vi "BuildRelease.vi"() -> ()   [LabVIEW 2014]
uses:
  <vilib>/Utility/traverseref.llb/TRef TravTarget.ctl
  <vilib>/Utility/traverseref.llb/VI Scripting - Traverse.lvlib
panel:
  out "error out":errorcluster
  out "Tab":enum32{"Start", "Building"}(tab)
  in  "Package Build":i32
  in  "AutoInstallAfterBuild":bool
  in  "DeleteRelease":bool
  in  "Output Folder":path=path "C:/OpenGDS" caption="Build folder: C:\\OpenGDS\\1.2.1(Master)"
  in  "LV_Versions":cluster{"LvVersion":string, "Check":bool}[](array[cluster]) caption="LV versions to compile the release for"
  in  "Build":bool
  out "Branch Name":string
  in  "New Version Number":string
  out "Current Version Number":string
  out "Progress":u8(slide) scale=0.0..100.0
  out "Progress":string
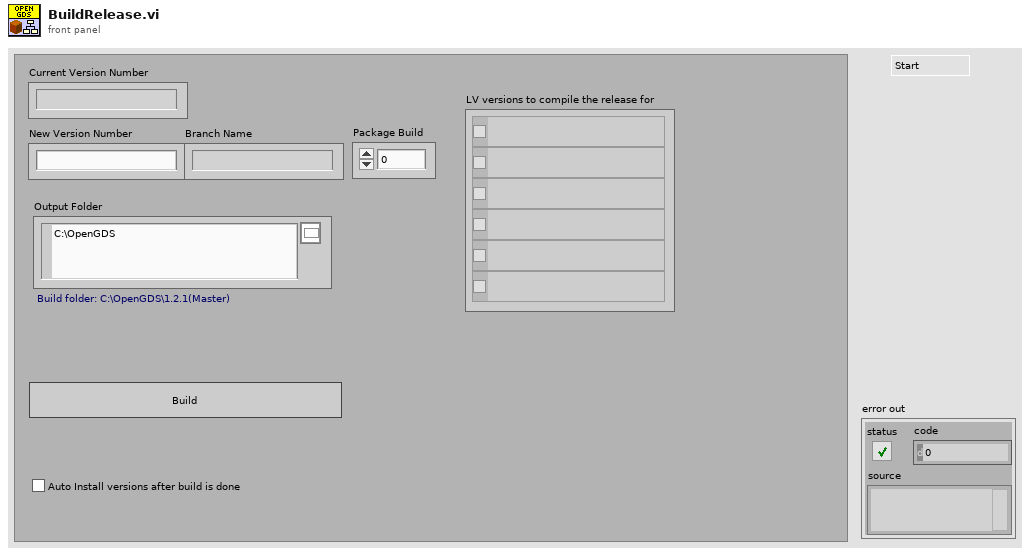
[diagram p1: front panel]
types:
  T1 = cluster{"LvVersion":path[], "BuildPath":path, "SourceFiles":path[], "LvVersion":string[], "SpecFile":path, "IniFiles":path[], "InstallerCopy":path, "VersionName":string, "InstallerFile":path, "ReadMeFile":path, "VIP-File":path, "LogFolder":path}
  T2 = enum32{"invalid OS target", "Mac OS", "Windows 3.1", "Windows 95/NT", "Solaris 1", "Solaris 2", "HP-UX", "PowerMAX", "Linux", "Irix", "Rhapsody", "BeOS", "AIX", "OSF1", "VxWorks", "PharLap", "Carbon", "RTX", "Windows x64", "Linux x64"}
  T3 = enum8{"Enabled", "Disabled", "Disabled and Grayed Out"}
  T4 = typedef "TRef TravTarget.ctl" = enum16{"FP", "BD", "Other"}
  T5 = enum32{"invalid OS target", "Mac OS", "Windows 3.1", "Windows 95/NT", "Solaris 1", "Solaris 2", "HP-UX", "PowerMAX", "Linux", "Irix", "Rhapsody", "BeOS", "AIX", "OSF1", "VxWorks", "PharLap", "Carbon", "RTX", "Windows x64", "Linux x64", "Mac OS X x64"}
  T6 = enum32{"not a typedef", "typedef", "strict typedef", "class private data"}
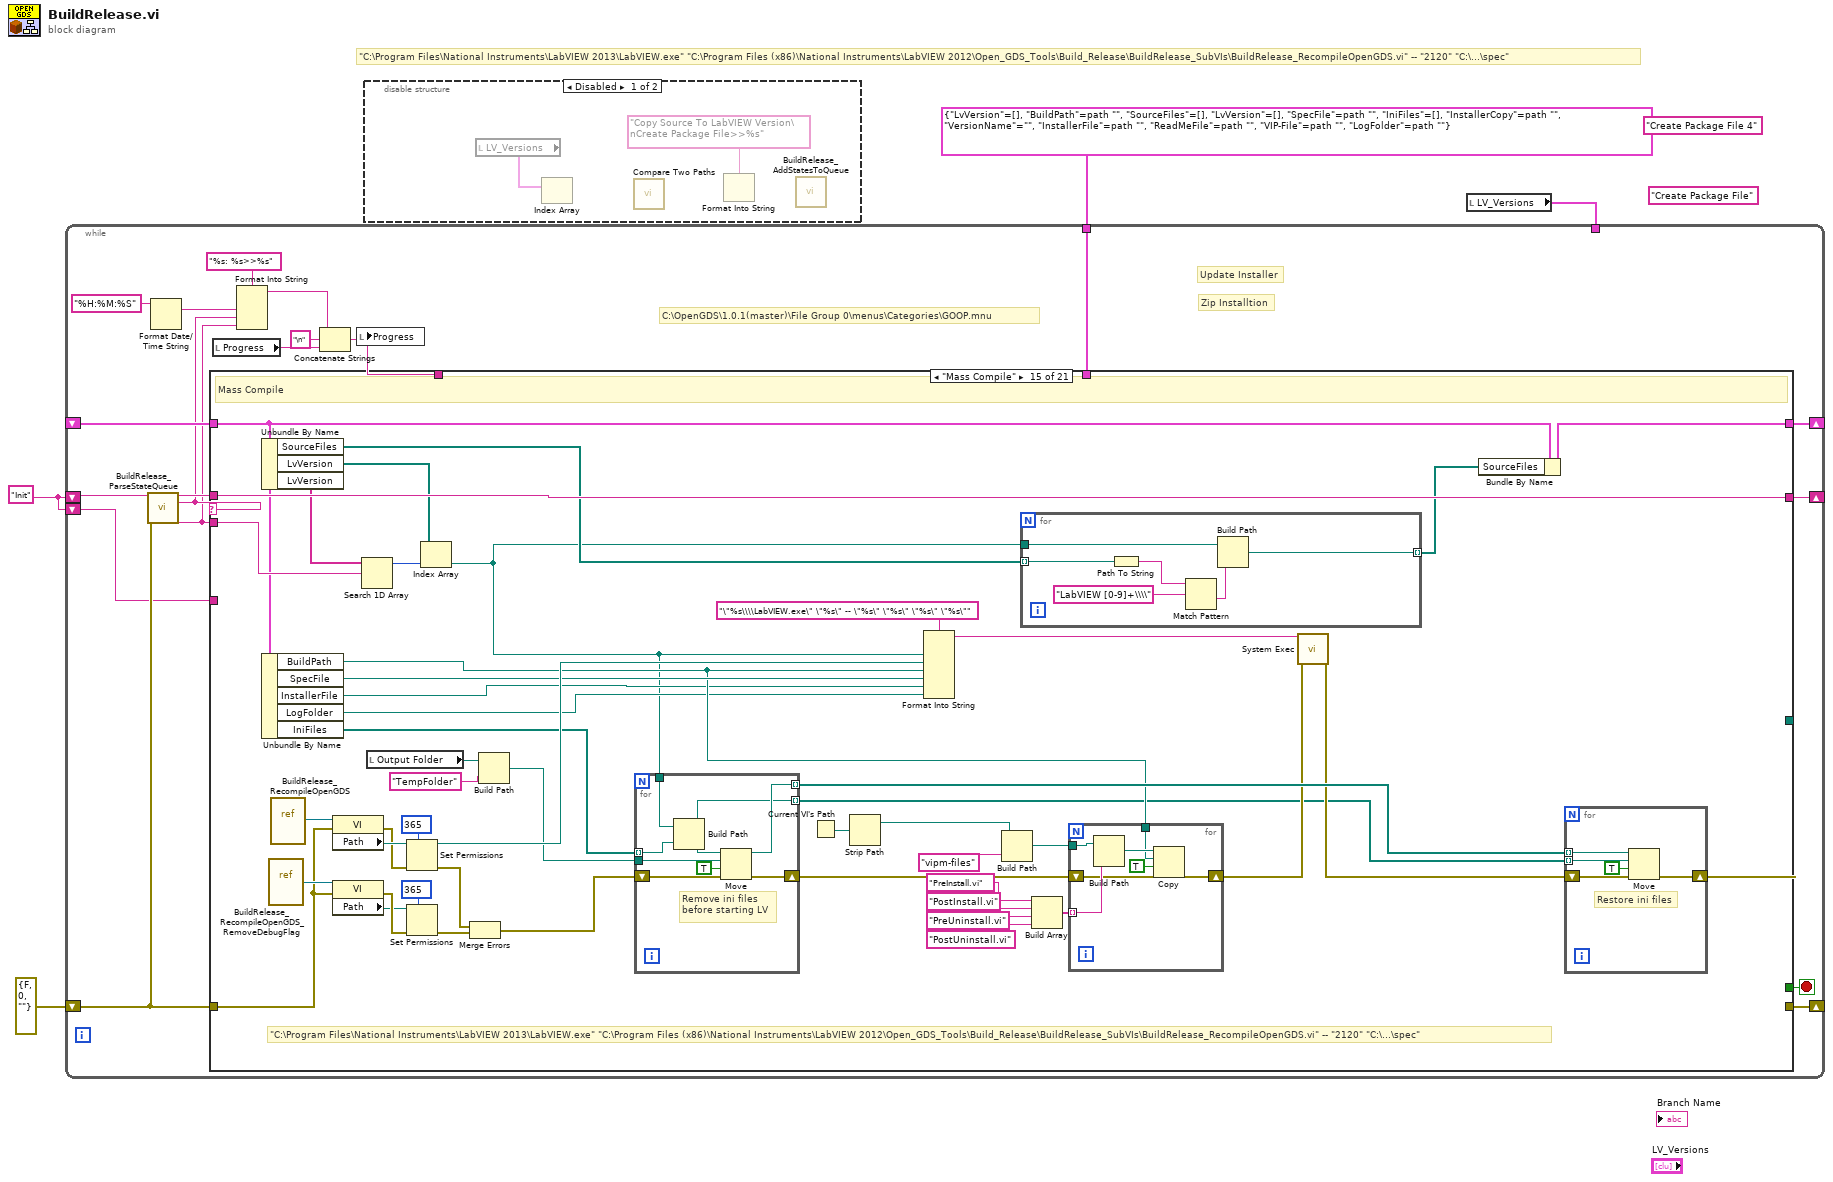
[diagram p0: block diagram]
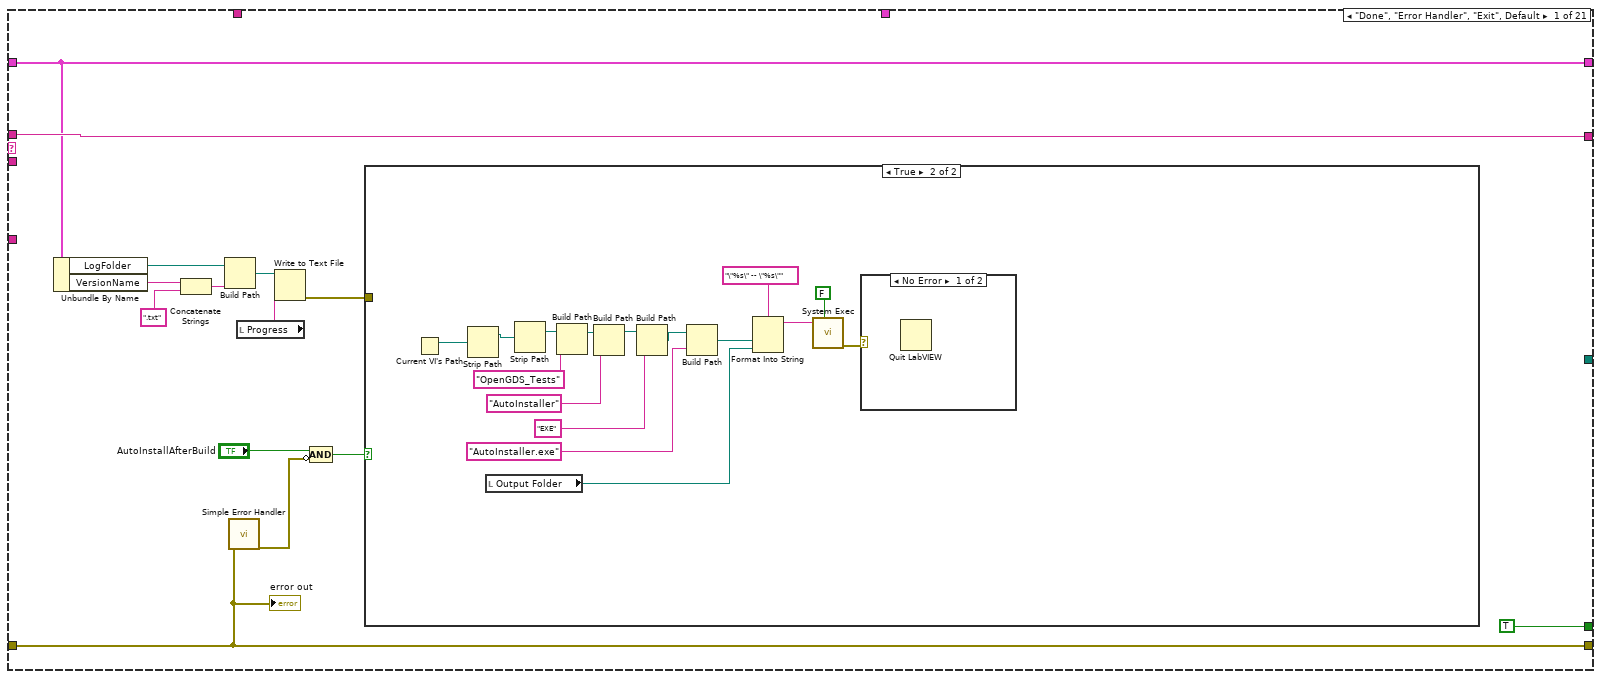
[diagram p3: hidden frame]
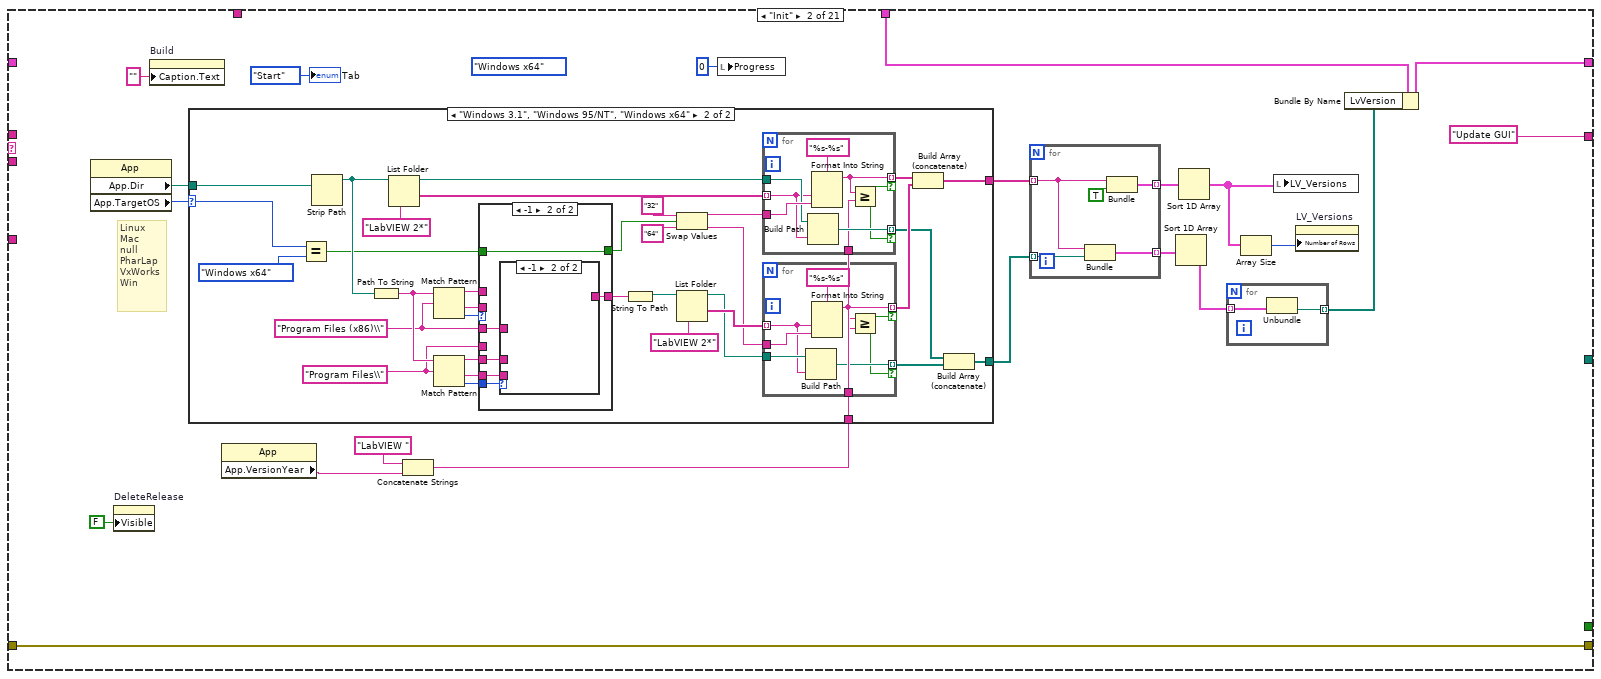
[diagram p6: hidden frame]
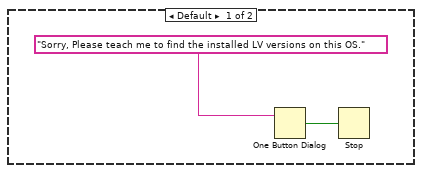
[diagram p7: hidden frame]
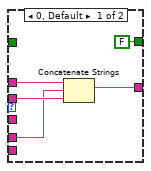
[diagram p8: hidden frame]
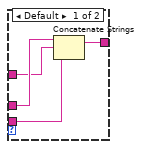
[diagram p9: hidden frame]
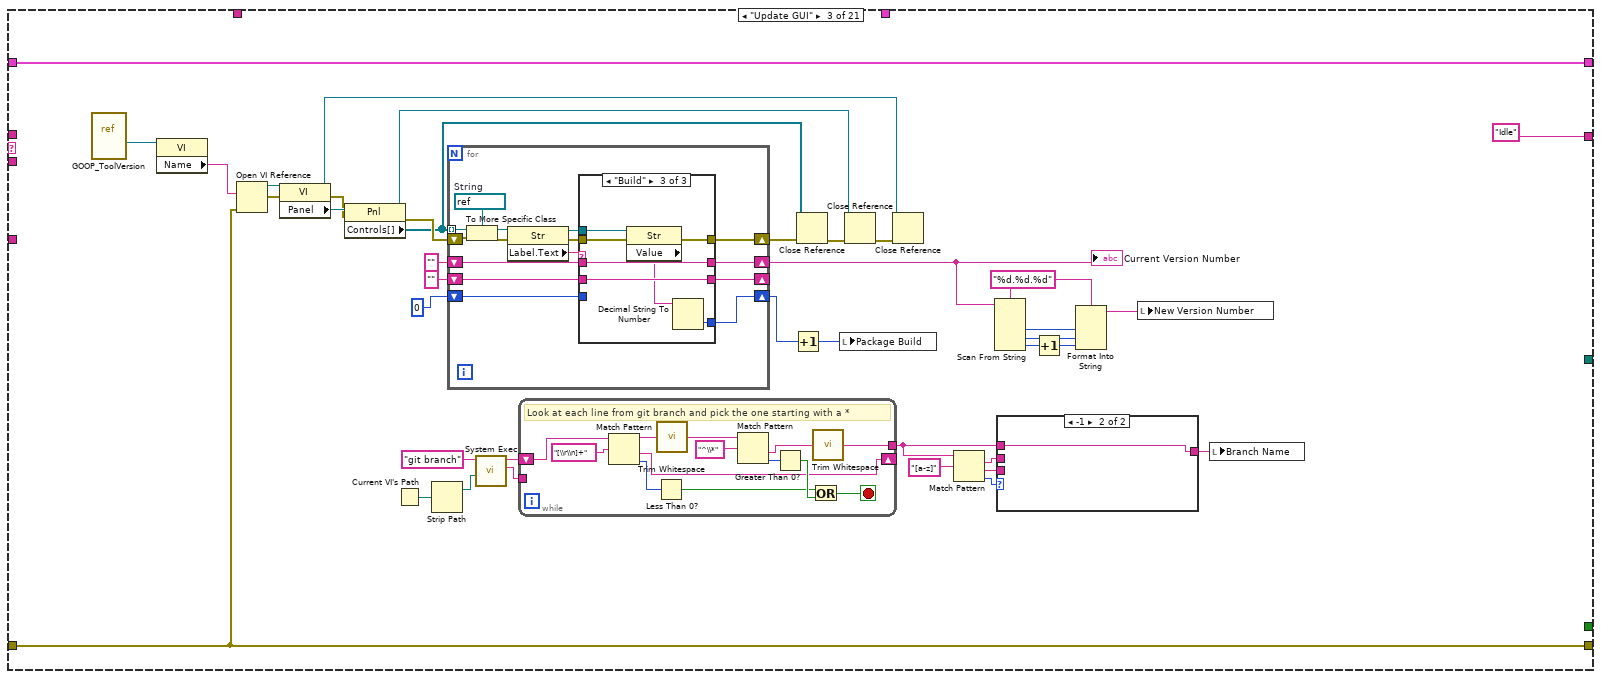
[diagram p10: hidden frame]
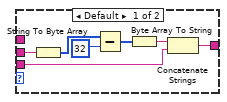
[diagram p11: hidden frame]
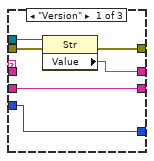
[diagram p12: hidden frame]
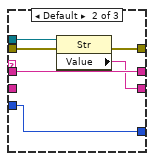
[diagram p13: hidden frame]
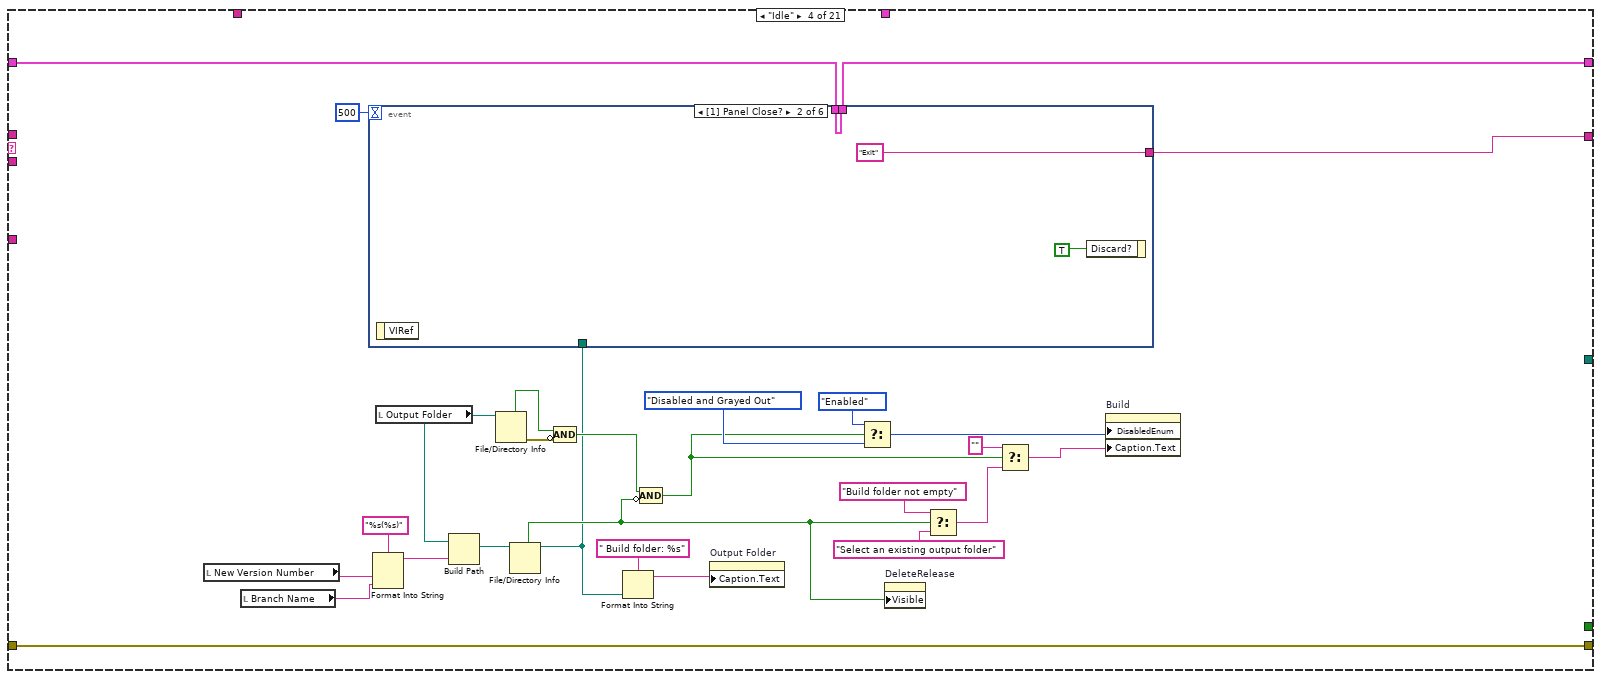
[diagram p14: hidden frame]
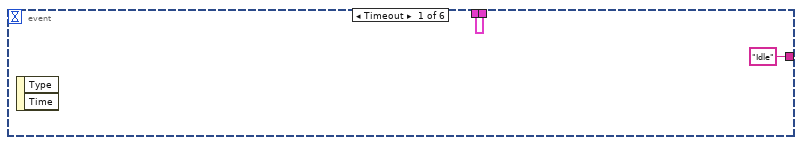
[diagram p15: hidden frame]
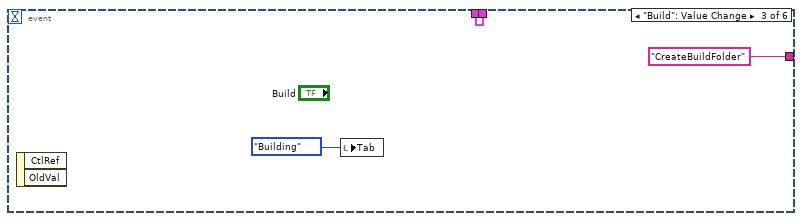
[diagram p16: hidden frame]
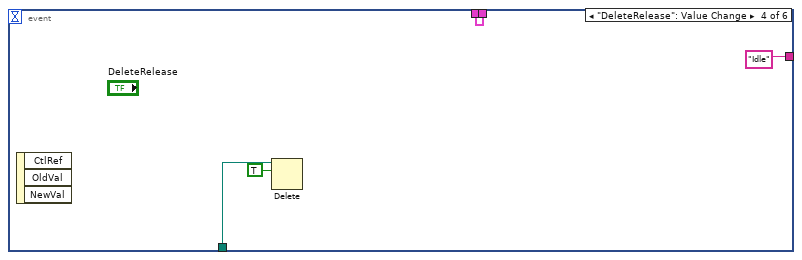
[diagram p17: hidden frame]
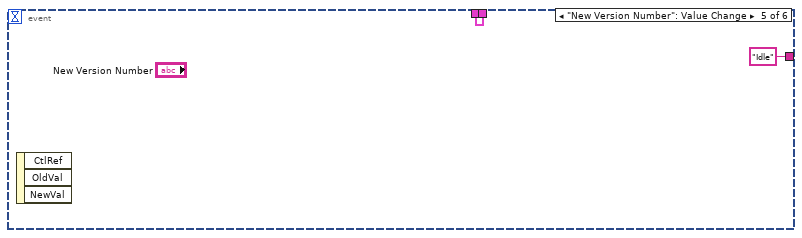
[diagram p18: hidden frame]
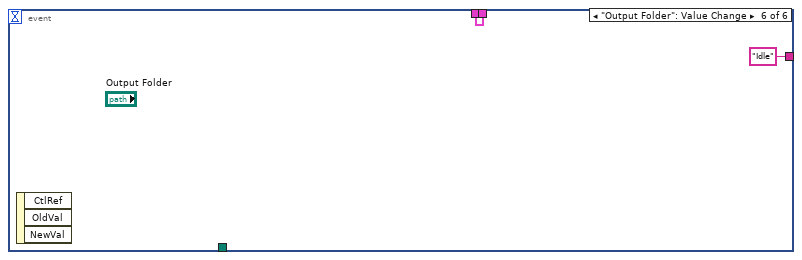
[diagram p19: hidden frame]
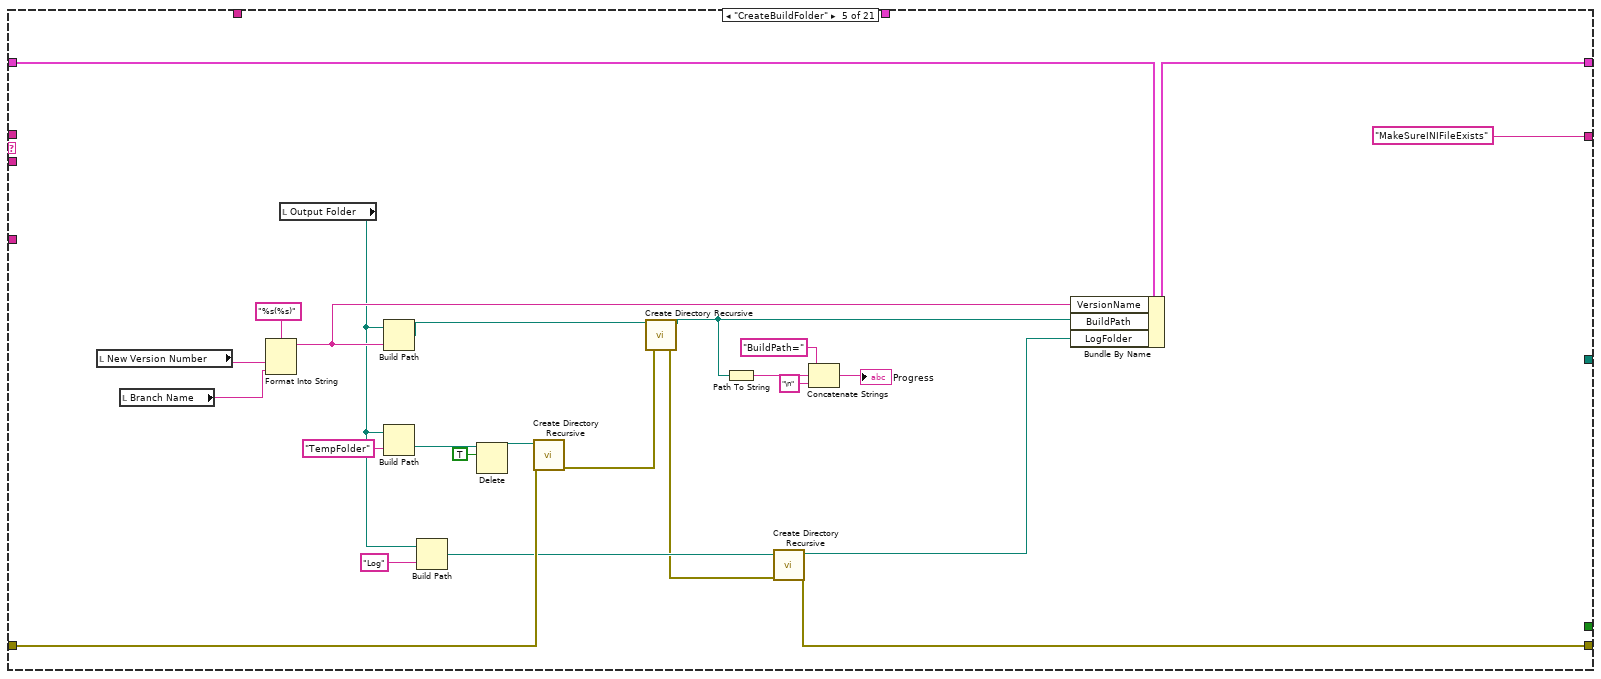
[diagram p20: hidden frame]
diagram:
  (unwired) "Create Package File 4"
  (unwired) "Create Package File"
  w1 = "Init"
  # "\"C:\\Program Files\\National Instruments\\LabVIEW 2013\\LabVIEW.exe\" \"C:\\Program Files (x86)\\National Instruments\\LabVIEW 2012\\Open_GDS_Tools\\Build_Release\\BuildRelease_SubVIs\\BuildRelease_RecompileOpenGDS.vi\" -- \"2120\" \"C:\\...\\spec\""
  n1 = disable-structure shown="Disabled" {
    frame Disabled {
      n2 = local read "LV_Versions"() -> (w5:cluster{"LvVersion":string, "Check":bool}[])
      n3 = Index Array(array=w5) -> ()  [unwired: 1 in, 1 out]
      n4 = call <vilib>:"Compare Two Paths.vi"() -> ()  [unwired: 8 in, 4 out]
      n5 = Format Into String(format string="Copy Source To LabVIEW Version\nCreate Package File>>%s") -> ()  [unwired: 3 in, 2 out]
      n6 = call "BuildRelease_AddStatesToQueue.vi"() -> ()  [unwired: 15 in, 1 out]
    }
    frame Enabled {
    }
  }
  n7 = local read "LV_Versions"() -> (w2:cluster{"LvVersion":string, "Check":bool}[])
  n8 = while {
    shift-right: [w25] -> _
    shift-left: errorcluster {"status"=FALSE, "code"=0, "source"=""} ("error IO") -> [w19]
    shift-right: [w18] -> _
    shift-left: w1 -> [w21]
    shift-right: [w24] -> _
    shift-left: _ -> [w23]
    tunnel: T1 {"LvVersion"=[], "BuildPath"=path "", "SourceFiles"=[], "LvVersion"=[], "SpecFile"=path "", "IniFiles"=[], "InstallerCopy"=path "", "VersionName"="", "InstallerFile"=path "", "ReadMeFile"=path "", "VIP-File"=path "", "LogFolder"=path ""} -> [w22]
    tunnel: w2 -> [_]
    shift-left: w1 -> [w7]
    stop <- w17 stop-if-true
    # "Zip Installtion"
    # "Update Installer"
    # "C:\\OpenGDS\\1.0.1(master)\\File Group 0\\menus\\Categories\\GOOP.mnu"
    n9 = call "BuildRelease_ParseStateQueue.vi"("State Queue"=w21, "Error In (no error)"=w19) -> ("Remaining States"=w20:string, "Current State"=w13:string, "Arguments"=w12:string)  [unwired: 11 in]
    n10 = Format Date/Time String(time format string (%c)="%H:%M:%S") -> (date/time string=w8:string)  [unwired: 2 in]
    n11 = local read "Progress"() -> (w15:string)
    n12 = Format Into String(format string="%s: %s>>%s", w8, w13, w12) -> (resulting string=w11:string)  [unwired: 2 in, 1 out]
    n13 = Concatenate Strings(w11, "\n" ("string"), w15) -> (w14:string)
    n14 = case shown="\"Mass Compile\"" w13 {
      tunnel: w19 -> [w26 w76 w172 w269 w297 w314 w354 w409 w490 w501 w560 w611 w632 w674 w729 w818 w836 w889 w911 w923 w964]
      tunnel: [w26 w76 w172 w269 w289 w313 w341 w397 w483 w500 w561 w611 w632 w658 w756 w803 w835 w877 w910 w930 w964] -> w25
      tunnel: [w37 w75 w189 w270 w308 w327 w340 w393 w492 w504 w559 w603 w631 w657 w755 w819 w826 w872 w913 w920 w963] -> w24
      tunnel: w23 -> [w37 _ w189 w271 w312 w327 w340 w412 w492 w504 w584 w609 w631 w680 w764 w819 w826 w890 w918 w920 w963]
      tunnel: w22 -> [_ w74 _ _ _ _ _ _ _ _ _ _ _ _ _ _ _ _ _ _ _]
      tunnel: w20 -> [w39 _ _ _ _ _ _ _ _ _ _ _ w630 w679 w776 w824 w834 w888 w917 w938 w962]
      tunnel: [w39 "Update GUI" "Idle" w247 "MakeSureINIFileExists" "Update Version Global VI" "Create Package File Spec File" "Add Package Extra Files" "Copy Source To LabVIEW Versions" "Copy Installer VI to Build Folder" "Create Build Process" w604 w630 w679 w776 w824 w834 w888 w917 w938 w962] -> w18
      tunnel: [TRUE _ _ _ _ _ _ _ _ _ _ _ _ _ _ _ _ _ _ _ _] -> w17
      tunnel: w12 -> [_ _ _ _ _ _ _ _ _ _ _ _ _ w633 w774 w822 w830 w879 w906 w932 _]
      tunnel: w14 -> [_ _ _ _ _ _ _ _ _ _ _ _ _ _ _ _ _ _ _ _ _]
      tunnel: w7 -> [_ _ _ _ _ _ _ _ _ _ _ _ _ _ _ _ _ _ _ _ _]
      tunnel: [_ _ _ _ _ _ _ _ _ _ _ _ _ _ _ _ w825 _ _ _ _] -> _
      frame "Done", "Error Handler", "Exit", Default {
        n15 = Unbundle By Name(w37) -> ("LogFolder"=w36:path, "VersionName"=w33:string)
        n16 = Concatenate Strings(w33, ".txt" ("format string")) -> (w32:string)
        n17 = Build Path(base path=w36, name or relative path=w32) -> (appended path=w35:path)
        n18 = call <vilib>:"Simple Error Handler.vi"("error in (no error)"=w26) -> ("error out"=w28:errorcluster)  [unwired: 4 in, 4 out]
        n19 = local read "Progress"() -> (w34:string)
        n20 = Write to Text File(file (use dialog)=w35, text=w34) -> (error out=w27:errorcluster)  [unwired: 2 in, 2 out]
        n21 = Compound Arithmetic op=AND("AutoInstallAfterBuild", invert w28) -> (w29:bool)
        n22 = case shown="True" w29 {
          tunnel: w27 -> [_ _]
          frame False {
          }
          frame True {
            n23 = Current VI's Path() -> (path=w53:path)
            n24 = Strip Path(path=w53) -> (stripped path=w52:path)  [unwired: 1 out]
            n25 = local read "Output Folder"() -> (w42:path)
            n26 = Strip Path(path=w52) -> (stripped path=w51:path)  [unwired: 1 out]
            n27 = Build Path(base path=w51, name or relative path="OpenGDS_Tests") -> (appended path=w49:path)
            n28 = Build Path(base path=w49, name or relative path="AutoInstaller") -> (appended path=w47:path)
            n29 = Build Path(base path=w47, name or relative path="EXE") -> (appended path=w45:path)
            n30 = Build Path(base path=w45, name or relative path="AutoInstaller.exe") -> (appended path=w43:path)
            n31 = Format Into String(format string="\"%s\" -- \"%s\"", w43, w42) -> (resulting string=w54:string)  [unwired: 2 in, 1 out]
            n32 = call <vilib>:"System Exec.vi"("wait until completion? (T)"=FALSE, "command line"=w54) -> ("error out"=w40:errorcluster)  [unwired: 6 in, 3 out]
            n33 = case shown="No Error" w40 {
              frame No Error {
                n34 = Quit LabVIEW() -> ()  [unwired: 1 in]
              }
              frame Error {
              }
            }
          }
        }
        "error out" <- w26
      }
      frame "Init" {
        (unwired) T2."Windows x64" ("y")
        # "Linux\nMac\nnull\nPharLap\nVxWorks\nWin"
        n35 = property class="App"() -> ("App.Dir"=w67:path, "App.TargetOS"=w68:T5)  [unwired: 2 in, 2 out]
        n36 = property on="DeleteRelease" class="Bool"("Visible"=FALSE) -> ()  [unwired: 2 in, 2 out]
        n37 = property on="Build" class="Bool"("Caption.Text"="") -> ()  [unwired: 2 in, 2 out]
        n38 = property class="App"() -> ("App.VersionYear"=w65:string)  [unwired: 2 in, 2 out]
        n39 = Concatenate Strings("LabVIEW " ("pattern"), w65) -> (w64:string)
        n40 = case shown="\"Windows 3.1\", \"Windows 95/NT\", \"Windows x64\"" w68 {
          selector: w68 -> [_ w82]
          tunnel: [_ w114] -> w73
          tunnel: w64 -> [_ w113]
          tunnel: [_ w112] -> w60
          tunnel: w67 -> [_ w81]
          frame Default {
            n41 = One Button Dialog(message="Sorry, Please teach me to find the installed LV versions on this OS.") -> (true=w79:bool)  [unwired: 1 in]
            n42 = Stop(stop? (T)=w79) -> ()
          }
          frame "Windows 3.1", "Windows 95/NT", "Windows x64" {
            w105 = "Program Files\\" ("regular expression")
            w90 = "Program Files (x86)\\" ("regular expression")
            n43 = Equal?(x=w82, y=T2."Windows x64") -> (x = y?=w93:bool)
            n44 = Strip Path(path=w81) -> (stripped path=w108:path)  [unwired: 1 out]
            n45 = Path To String(path=w108) -> (string=w110:string)
            n46 = List Folder(path=w108, pattern="LabVIEW 2*") -> (path out=w84:path, folder names=w101:string[])  [unwired: 2 in, 2 out]
            n47 = Match Pattern(string=w110, regular expression=w90) -> (before substring=w107:string, after substring=w106:string, offset past match=w109:i32)  [unwired: 1 in, 1 out]
            n48 = Match Pattern(string=w110, regular expression=w105) -> (before substring=w92:string, after substring=w91:string, offset past match=w95:i32)  [unwired: 1 in, 1 out]
            n49 = case shown="-1" w109 {
              tunnel: w107 -> [w135 _]
              tunnel: w106 -> [w134 _]
              tunnel: w105 -> [w133 _]
              tunnel: [w132 w136] -> w104
              tunnel: [FALSE w140] -> w100
              tunnel: w95 -> [_ w141]
              tunnel: w93 -> [_ w140]
              tunnel: w92 -> [_ w139]
              tunnel: w91 -> [_ w138]
              tunnel: w90 -> [_ w137]
              frame 0, Default {
                n50 = Concatenate Strings(w135, w133, w134) -> (w132:string)
              }
              frame -1 {
                n51 = case shown="-1" w141 {
                  tunnel: w139 -> [w145 _]
                  tunnel: w138 -> [w144 _]
                  tunnel: w137 -> [w143 _]
                  tunnel: [w142 _] -> w136
                  frame Default {
                    n52 = Concatenate Strings(w145, w143, w144) -> (w142:string)
                  }
                  frame -1 {
                  }
                }
              }
            }
            n53 = String To Path(string=w104) -> (path=w102:path)
            n54 = Swap Values(12:"32" ("format string"), 13:w100, 14:"64" ("format string")) -> (1:w97:string, 3:w87:string)
            n55 = List Folder(path=w102, pattern="LabVIEW 2*") -> (path out=w86:path, folder names=w96:string[])  [unwired: 2 in, 2 out]
            n56 = for {
              tunnel: w101 -> [w127] mode=indexing
              tunnel: w97 -> [w129]
              tunnel: [w125] -> w89 mode=indexing if=w123
              tunnel: w84 -> [w128]
              tunnel: [w126] -> w83 mode=indexing if=w123
              tunnel: w113 -> [w124]
              n57 = Build Path(base path=w128, name or relative path=w127) -> (appended path=w126:path)
              n58 = Format Into String(format string="%s-%s", w127, w129) -> (resulting string=w125:string)  [unwired: 2 in, 1 out]
              n59 = Greater Or Equal?(x=w125, y=w124) -> (x >= y?=w123:bool)
            }
            n60 = for {
              tunnel: w96 -> [w119] mode=indexing
              tunnel: w87 -> [w121]
              tunnel: [w117] -> w88 mode=indexing if=w115
              tunnel: w86 -> [w120]
              tunnel: [w118] -> w85 mode=indexing if=w115
              tunnel: w113 -> [w116]
              n61 = Build Path(base path=w120, name or relative path=w119) -> (appended path=w118:path)
              n62 = Format Into String(format string="%s-%s", w119, w121) -> (resulting string=w117:string)  [unwired: 2 in, 1 out]
              n63 = Greater Or Equal?(x=w117, y=w116) -> (x >= y?=w115:bool)
            }
            n64 = Build Array (concatenate)(w89, w88) -> (w114:string[])
            n65 = Build Array (concatenate)(w83, w85) -> (w112:path[])
          }
        }
        n66 = local write "Progress"(u8 0 ("Progress")) -> ()
        n67 = for {
          tunnel: w73 -> [w149] mode=indexing
          tunnel: [w150] -> w72 mode=indexing
          tunnel: w60 -> [w148] mode=indexing
          tunnel: [w147] -> w58 mode=indexing
          n68 = Bundle(w149, "appended path"=w148) -> (w147:cluster{string, "appended path":path})  [unwired: 1 in]
          n69 = Bundle(w149, "Check"=TRUE) -> (w150:cluster{string, "Check":bool})  [unwired: 1 in]
        }
        n70 = Sort 1D Array(array=w58) -> (sorted array=w57:cluster{string, "appended path":path}[])
        n71 = Sort 1D Array(array=w72) -> (sorted array=w59:cluster{string, "Check":bool}[])
        n72 = for {
          tunnel: w57 -> [w78] mode=indexing
          tunnel: [w77] -> w56 mode=indexing
          n73 = Unbundle(w78) -> ("appended path"=w77:path)  [unwired: 1 out]
        }
        n74 = Array Size(array=w59) -> (size(s)=w71:i32)
        n75 = local write "LV_Versions"(w59) -> ()
        n76 = property on="LV_Versions" class="Arr (strict)"("Number of Rows"=w71) -> ()  [unwired: 2 in, 2 out]
        n77 = Bundle By Name(cluster=w74, "LvVersion"=w56) -> (w75:T1)
        "Tab" <- enum32{"Start", "Building"}."Start" ("Tab")
      }
      frame "Update GUI" {
        w188 = "%d.%d.%d" ("format string")
        n78 = vi-ref <resource>:"GOOP_ToolVersion.vi"() -> (w179:refnum<vi>)
        n79 = property class="VI"(reference=w179) -> ("Name"=w178:string)  [unwired: 1 in, 2 out]
        n80 = Open VI Reference(vi path=w178, error in (no error)=w172) -> (vi reference=w177:refnum<vi>, error out=w176:errorcluster)  [unwired: 4 in]
        n81 = property class="VI"(reference=w177, error in=w176) -> (reference out=w166:refnum<vi>, error out=w173:errorcluster, "Panel"=w175:refnum<vi>)
        n82 = property class="Pnl"(reference=w175, error in=w173) -> (reference out=w168:refnum<vi>, error out=w174:errorcluster, "Controls[]"=w170:refnum<vi>[])
        n83 = Current VI's Path() -> (path=w182:path)
        n84 = Strip Path(path=w182) -> (stripped path=w181:path)  [unwired: 1 out]
        n85 = for {
          tunnel: w170 -> [w224] mode=indexing
          shift-right: [w220] -> w171
          shift-left: w174 -> [w217]
          shift-right: [w216] -> w163
          shift-left: "" ("Value") -> [w215]
          shift-right: [w214] -> _
          shift-left: "" ("Value") -> [w213]
          shift-right: [w211] -> w152
          shift-left: 0 -> [w212]
          w223 = refnum<vi> refnum  # String
          n86 = To More Specific Class(target class=w223, reference=w224, error in=w217) -> (specific class reference=w222:refnum<vi>, error out=w218:errorcluster)
          n87 = property class="Str"(reference=w222, error in=w218) -> (reference out=w221:refnum<vi>, error out=w219:errorcluster, "Label.Text"=w225:string)
          n88 = case shown="\"Build\"" w225 {
            tunnel: w221 -> [w231 w237 w244]
            tunnel: [w229 w236 w243] -> w220
            tunnel: w219 -> [w230 w235 w242]
            tunnel: [w228 w234 w241] -> w216
            tunnel: w215 -> [_ w234 w241]
            tunnel: [w227 w233 w240] -> w214
            tunnel: w213 -> [w227 _ w240]
            tunnel: w212 -> [w226 w232 _]
            tunnel: [w226 w232 w238] -> w211
            frame "Version" {
              n89 = property class="Str"(reference=w231, error in=w230) -> (error out=w229:errorcluster, "Value"=w228:string)  [unwired: 1 out]
            }
            frame Default {
              n90 = property class="Str"(reference=w237, error in=w235) -> (error out=w236:errorcluster, "Value"=w233:string)  [unwired: 1 out]
            }
            frame "Build" {
              n91 = property class="Str"(reference=w244, error in=w242) -> (error out=w243:errorcluster, "Value"=w239:string)  [unwired: 1 out]
              n92 = Decimal String To Number(string=w239) -> (number=w238:i32)  [unwired: 2 in, 1 out]
            }
          }
        }
        "Current Version Number" <- w163
        n93 = call <vilib>:"System Exec.vi"("working directory"=w181, "command line"="git branch") -> ("standard error"=w154:string, "standard output"=w155:string)  [unwired: 6 in, 2 out]
        n94 = while {
          tunnel: [w190] -> w156
          shift-right: [w193] -> _
          shift-left: w155 -> [w197]
          tunnel: w154 -> [_]
          stop <- w196 stop-if-true
          # "Look at each line from git branch and pick the one starting with a *"
          n95 = Match Pattern(string=w197, regular expression="[\\r\\n]+") -> (before substring=w194:string, after substring=w193:string, offset past match=w195:i32)  [unwired: 1 in, 1 out]
          n96 = Less Than 0?(x=w195) -> (x < 0?=w191:bool)
          n97 = call <vilib>:"Trim Whitespace.vi"("string"=w194) -> ("trimmed string"=w202:string)  [unwired: 1 in]
          n98 = Match Pattern(string=w202, regular expression="^\\*") -> (after substring=w200:string, offset past match=w199:i32)  [unwired: 1 in, 2 out]
          n99 = Greater Than 0?(x=w199) -> (x > 0?=w198:bool)
          n100 = Or(x=w191, y=w198) -> (x .or. y?=w196:bool)
          n101 = call <vilib>:"Trim Whitespace.vi"("string"=w200) -> ("trimmed string"=w190:string)  [unwired: 1 in]
        }
        n102 = Increment(x=w152) -> (x+1=w151:i32)
        n103 = Close Reference(reference=w170, error in (no error)=w171) -> (error out=w169:errorcluster)
        n104 = local write "Package Build"(w151) -> ()
        n105 = Close Reference(reference=w168, error in (no error)=w169) -> (error out=w167:errorcluster)
        n106 = Close Reference(reference=w166, error in (no error)=w167) -> ()  [unwired: 1 out]
        n107 = Match Pattern(string=w156, regular expression="[a-z]") -> (match substring=w158:string, after substring=w157:string, offset past match=w160:i32)  [unwired: 1 in, 1 out]
        n108 = Scan From String(format string=w188, input string=w163) -> (output 1=w187:i32, output 2=w186:i32, output 3=w185:i32)  [unwired: 5 in, 3 out]
        n109 = case shown="-1" w160 {
          tunnel: w156 -> [_ w210]
          tunnel: [w203 w210] -> w159
          tunnel: w158 -> [w209 _]
          tunnel: w157 -> [w204 _]
          frame Default {
            n110 = String To Byte Array(string=w209) -> (unsigned byte array=w208:u8[])
            n111 = Subtract(x=w208, y=32) -> (x-y=w206:i32[])
            n112 = Byte Array To String(unsigned byte array=w206) -> (string=w205:string)
            n113 = Concatenate Strings(w205, w204) -> (w203:string)
          }
          frame -1 {
          }
        }
        n114 = Increment(x=w185) -> (x+1=w184:i32)
        n115 = Format Into String(format string=w188, w187, w186, w184) -> (resulting string=w183:string)  [unwired: 2 in, 1 out]
        n116 = local write "New Version Number"(w183) -> ()
        n117 = local write "Branch Name"(w159) -> ()
      }
      frame "Idle" {
        n118 = local read "New Version Number"() -> (w260:string)
        n119 = local read "Branch Name"() -> (w261:string)
        n120 = Format Into String(format string="%s(%s)", w260, w261) -> (resulting string=w258:string)  [unwired: 2 in, 1 out]
        n121 = local read "Output Folder"() -> (w256:path)
        n122 = Build Path(base path=w256, name or relative path=w258) -> (appended path=w257:path)
        n123 = File/Directory Info(path=w256) -> (directory=w267:bool, error out=w268:errorcluster)  [unwired: 1 in, 5 out]
        n124 = File/Directory Info(path=w257) -> (path out=w245:path, directory=w246:bool)  [unwired: 1 in, 5 out]
        n125 = event shown="[1] Panel Close?" {
          selector: _ -> [_ _ _ _ _ _]
          dyn-events: _ -> [_ _ _ _ _ _]
          timeout: 500 -> [_ _ _ _ _ _]
          tunnel: w271 -> [w273 w275 w279 w283 w285 w287]
          tunnel: [w273 w275 w279 w283 w285 w287] -> w270
          tunnel: ["Idle" "Exit" "CreateBuildFolder" "Idle" "Idle" "Idle"] -> w247
          tunnel: w245 -> [_ _ _ w282 _ _]
          event Timeout {
            n126 = event-data() -> ()  [unwired: 1 in, 2 out]
          }
          event Panel Close? {
            n127 = event-data() -> ()  [unwired: 1 in, 1 out]
            n128 = event-data("Discard?"=TRUE) -> ()  [unwired: 1 in, 1 out]
          }
          event "Build": Value Change {
            n129 = event-data() -> ()  [unwired: 1 in, 2 out]
            n130 = local write "Tab"(enum32{"Start", "Building"}."Building" ("Tab")) -> ()
          }
          event "DeleteRelease": Value Change {
            n131 = event-data() -> ()  [unwired: 1 in, 3 out]
            n132 = Delete(path (use dialog)=w282, entire hierarchy (F)=TRUE) -> ()  [unwired: 3 in, 3 out]
          }
          event "New Version Number": Value Change {
            n133 = event-data() -> ()  [unwired: 1 in, 3 out]
          }
          event "Output Folder": Value Change {
            n134 = event-data() -> ()  [unwired: 1 in, 3 out]
          }
        }
        n135 = Compound Arithmetic op=AND(w267, invert w268) -> (w254:bool)
        n136 = Format Into String(format string=" Build folder: %s", w245) -> (resulting string=w249:string)  [unwired: 2 in, 1 out]
        n137 = Compound Arithmetic op=AND(w254, invert w246) -> (w255:bool)
        n138 = property on="Output Folder" class="Path"("Caption.Text"=w249) -> ()  [unwired: 2 in, 2 out]
        n139 = Select(t=T3."Enabled" ("Disabled"), s=w255, f=T3."Disabled and Grayed Out" ("Disabled")) -> (s? t:f=w266:T3)
        n140 = property on="DeleteRelease" class="Bool"("Visible"=w246) -> ()  [unwired: 2 in, 2 out]
        n141 = Select(t="Build folder not empty" ("Caption.Text"), s=w246, f="Select an existing output folder" ("Caption.Text")) -> (s? t:f=w251:string)
        n142 = Select(t="" ("Caption.Text"), s=w255, f=w251) -> (s? t:f=w262:string)
        n143 = property on="Build" class="Bool"("DisabledEnum"=w266, "Caption.Text"=w262) -> ()  [unwired: 2 in, 2 out]
      }
      frame "CreateBuildFolder" {
        n144 = local read "New Version Number"() -> (w310:string)
        n145 = local read "Branch Name"() -> (w311:string)
        n146 = Format Into String(format string="%s(%s)", w310, w311) -> (resulting string=w294:string)  [unwired: 2 in, 1 out]
        n147 = local read "Output Folder"() -> (w293:path)
        n148 = Build Path(base path=w293, name or relative path=w294) -> (appended path=w300:path)
        n149 = Build Path(base path=w293, name or relative path="TempFolder") -> (appended path=w302:path)
        n150 = Build Path(base path=w293, name or relative path="Log") -> (appended path=w291:path)
        n151 = Delete(path (use dialog)=w302, entire hierarchy (F)=TRUE) -> (deleted path=w298:path)  [unwired: 3 in, 2 out]
        n152 = call <vilib>:"Create Directory Recursive.vi"("error in (no error)"=w297, "directory"=w298) -> ("error out"=w296:errorcluster)  [unwired: 3 in, 2 out]
        n153 = call <vilib>:"Create Directory Recursive.vi"("error in (no error)"=w296, "directory"=w300) -> ("error out"=w290:errorcluster, "directory copy"=w299:path)  [unwired: 3 in, 1 out]
        n154 = Path To String(path=w299) -> (string=w306:string)
        n155 = call <vilib>:"Create Directory Recursive.vi"("error in (no error)"=w290, "directory"=w291) -> ("error out"=w289:errorcluster, "directory copy"=w288:path)  [unwired: 3 in, 1 out]
        n156 = Concatenate Strings("BuildPath=" ("string"), w306, "\n" ("string")) -> (→"Progress":string)
        n157 = Bundle By Name(cluster=w312, "VersionName"=w294, "BuildPath"=w299, "LogFolder"=w288) -> (w308:T1)
      }
      frame "MakeSureINIFileExists" {
        # "INI-FILES-GProviders"
        n158 = property class="App"() -> ("App.Dir"=w317:path)  [unwired: 2 in, 2 out]
        n159 = Current VI's Path() -> (path=w325:path)
        n160 = Strip Path(path=w325) -> (stripped path=w324:path)  [unwired: 1 out]
        n161 = Strip Path(path=w324) -> (stripped path=w323:path)  [unwired: 1 out]
        n162 = for {
          shift-right: [w329] -> w315
          shift-left: w317 -> [w330]
          tunnel: string[] ["resource", "Framework", "Providers", "GProviders"] -> [w328] mode=indexing
          n163 = Build Path(base path=w330, name or relative path=w328) -> (appended path=w329:path)
        }
        n164 = Build Path(base path=w323, name or relative path="INI-FILES-GProviders" ("string")) -> (appended path=w321:path)
        n165 = call <vilib>:"Recursive File List.vi"("pattern"="*.ini", "error in (no error)"=w314, "Folder Path"=w321) -> ("error out"=w318:errorcluster, "All Files in Dir"=w319:path[])  [unwired: 4 in, 3 out]
        n166 = for {
          tunnel: w319 -> [w335] mode=indexing
          shift-right: [w331] -> w313
          shift-left: w318 -> [w334]
          tunnel: w315 -> [w332]
          n167 = Copy(8:w334, 9:TRUE ("overwrite (F)"), 10:w332, 11:w335) -> (0:w331:errorcluster)  [unwired: 1 in, 2 out]
        }
      }
      frame "Update Version Global VI" {
        n168 = vi-ref <resource>:"GOOP_ToolVersion.vi"() -> (w356:refnum<vi>)
        n169 = property class="VI"(reference=w356) -> ("Name"=w355:string)  [unwired: 1 in, 2 out]
        n170 = Open VI Reference(vi path=w355, error in (no error)=w354) -> (vi reference=w353:refnum<vi>, error out=w352:errorcluster)  [unwired: 4 in]
        n171 = property class="VI"(reference=w353, error in=w352) -> (reference out=w342:refnum<vi>, error out=w348:errorcluster, "Panel"=w351:refnum<vi>)
        n172 = property class="Pnl"(reference=w351, error in=w348) -> (error out=w349:errorcluster, "Controls[]"=w350:refnum<vi>[])  [unwired: 1 out]
        n173 = local read "New Version Number"() -> (w338:string)
        n174 = local read "Branch Name"() -> (w339:string)
        n175 = local read "Package Build"() -> (w336:i32)
        n176 = for {
          tunnel: w350 -> [w367] mode=indexing
          shift-right: [w363] -> w343
          shift-left: w349 -> [w360]
          tunnel: w338 -> [w359]
          tunnel: w339 -> [w358]
          tunnel: w336 -> [w357]
          w366 = refnum<vi> refnum  # String
          n177 = To More Specific Class(target class=w366, reference=w367, error in=w360) -> (specific class reference=w365:refnum<vi>, error out=w361:errorcluster)
          n178 = property class="Str"(reference=w365, error in=w361) -> (reference out=w364:refnum<vi>, error out=w362:errorcluster, "Label.Text"=w368:string)
          n179 = case shown="\"Build\"" w368 {
            tunnel: w364 -> [w372 w377 w381]
            tunnel: [w370 w375 w380] -> w363
            tunnel: w362 -> [w371 w376 w379]
            tunnel: w359 -> [w369 _ _]
            tunnel: w358 -> [_ _ w378]
            tunnel: w357 -> [_ w374 _]
            frame "Version" {
              n180 = property class="Str"(reference=w372, error in=w371, "Value"=w369) -> (error out=w370:errorcluster)  [unwired: 1 out]
            }
            frame "Build" {
              n181 = Number To Decimal String(number=w374) -> (decimal integer string=w373:string)  [unwired: 1 in]
              n182 = property class="Str"(reference=w377, error in=w376, "Value"=w373) -> (error out=w375:errorcluster)  [unwired: 1 out]
            }
            frame Default {
              n183 = property class="Str"(reference=w381, error in=w379, "Value"=w378) -> (error out=w380:errorcluster)  [unwired: 1 out]
            }
          }
        }
        n184 = invoke class="VI" method="Default Vals.Make Curr Default"(reference=w342, error in=w343) -> (reference out=w345:refnum<vi>, error out=w344:errorcluster)  [unwired: 1 in, 1 out]
        n185 = invoke class="VI" method="Save.Instrument"(reference=w345, error in=w344) -> (reference out=w346:refnum<vi>, error out=w347:errorcluster)  [unwired: 4 in, 4 out]
        n186 = Close Reference(reference=w346, error in (no error)=w347) -> (error out=w341:errorcluster)
      }
      frame "Create Package File Spec File" {
        # "Create The Spec file"
        n187 = Current VI's Path() -> (path=w430:path)
        n188 = Strip Path(path=w430) -> (stripped path=w416:path)  [unwired: 1 out]
        n189 = Build Path(base path=w416, name or relative path="OpenGDS_FileList.txt") -> (appended path=w426:path)
        n190 = Build Path(base path=w416, name or relative path="vipm-files") -> (appended path=w415:path)
        n191 = property class="App"() -> ("App.Dir"=w427:path)  [unwired: 2 in, 2 out]
        n192 = Read from Text File(file (use dialog)=w426, error in=w409) -> (text=w425:string, error out=w408:errorcluster)  [unwired: 2 in, 2 out]
        n193 = call <vilib>:"Trim Whitespace.vi"("string"=w425) -> ("trimmed string"=w424:string)  [unwired: 1 in]
        n194 = Build Path(base path=w415, name or relative path="vipm_spec_template.txt") -> (appended path=w419:path)
        n195 = Spreadsheet String To Array(delimiter (Tab)="\n", format string="%s", spreadsheet string=w424, array type (2D Dbl)=string[] []) -> (array=w420:string[])
        n196 = Read from Text File(file (use dialog)=w419, error in=w408) -> (text=w388:string, error out=w407:errorcluster)  [unwired: 2 in, 2 out]
        n197 = for {
          tunnel: w427 -> [w451]
          tunnel: w420 -> [w452] mode=indexing
          tunnel: [w446] -> w405 mode=concatenating
          n198 = Build Path(base path=w451, name or relative path=w452) -> (appended path=w450:path)
          n199 = File/Directory Info(path=w450) -> (path out=w447:path, directory=w448:bool, error out=w449:errorcluster)  [unwired: 1 in, 4 out]
          n200 = case shown="No Error" w449 {
            selector: w449 -> [w454 _]
            tunnel: w448 -> [w456 _]
            tunnel: w447 -> [w455 _]
            tunnel: [w453 _] -> w446
            frame No Error {
              n201 = case shown="False" w456 {
                tunnel: w455 -> [w458 w461]
                tunnel: w454 -> [_ w460]
                tunnel: [w457 w459] -> w453
                frame False {
                  n202 = Build Array(w458) -> (w457:path[])
                }
                frame True {
                  n203 = call <vilib>:"Recursive File List.vi"("error in (no error)"=w460, "Folder Path"=w461) -> ("All Files in Dir"=w459:path[])  [unwired: 5 in, 4 out]
                }
              }
            }
            frame Error {
            }
          }
        }
        n204 = local read "New Version Number"() -> (w386:string)
        n205 = Format Into String(format string=".%d", initial string=w386, "Package Build") -> (resulting string=w383:string)  [unwired: 1 in, 1 out]
        n206 = Search and Replace String(input string=w388, search string="<version>", replace string=w383) -> (result string=w389:string)  [unwired: 5 in, 3 out]
        n207 = Array Size(array=w405) -> (size(s)=w391:i32)
        n208 = stacked-sequence {
          tunnel: w391 -> [_]
          tunnel: [w431] -> w390
          frame #0 {
            n209 = Format Date/Time String(time format string (%c)="%H:%M: ") -> (date/time string=w431:string)  [unwired: 2 in]
          }
        }
        n210 = Bundle By Name(cluster=w412, "SourceFiles"=w405) -> (w406:T1)
        n211 = Format Into String(format string="%d\n", initial string=w389, w391) -> (resulting string=w417:string)  [unwired: 1 in, 1 out]
        n212 = Format Into String(format string="Files:%d", initial string=w390, w391) -> (resulting string=w399:string)  [unwired: 1 in, 1 out]
        n213 = local read "Progress"() -> (w402:string)
        n214 = for {
          tunnel: w405 -> [w439] mode=indexing
          shift-right: [w441] -> w394
          shift-left: w417 -> [w445]
          tunnel: [w434] -> w382 mode=indexing if=w433
          i -> [w443]
          n215 = Path To String(path=w439) -> (string=w440:string)
          n216 = Strip Path(path=w439) -> (name=w438:string)  [unwired: 1 out]
          n217 = Match Pattern(string=w440, regular expression="LabVIEW [0-9]+[\\\\/]") -> (after substring=w435:string)  [unwired: 1 in, 3 out]
          n218 = Match Pattern(string=w438, regular expression="^GOOP_[A-Za-z]+.ini$") -> (offset past match=w436:i32)  [unwired: 1 in, 3 out]
          n219 = Format Into String(format string="File %d=\"%s\"\n", initial string=w445, w443, w435) -> (resulting string=w441:string)  [unwired: 1 in, 1 out]
          n220 = String To Path(string=w435) -> (path=w434:path)
          n221 = Greater Or Equal To 0?(x=w436) -> (x >= 0?=w433:bool)
        }
        n222 = Concatenate Strings(w399, "\n" ("string"), w402) -> (w403:string)
        n223 = Unbundle By Name(w406) -> ("BuildPath"=w411:path)
        n224 = local write "Progress"(w403) -> ()
        n225 = Build Path(base path=w411, name or relative path="spec") -> (appended path=w410:path)
        n226 = Write to Text File(file (use dialog)=w410, text=w394, error in=w407) -> (error out=w398:errorcluster)  [unwired: 1 in, 2 out]
        n227 = local read "Output Folder"() -> (w395:path)
        n228 = Build Path(base path=w395, name or relative path="spec_File.txt") -> (appended path=w392:path)
        n229 = Bundle By Name(cluster=w406, "IniFiles"=w382, "SpecFile"=w392) -> (w393:T1)
        n230 = Write to Text File(file (use dialog)=w392, text=w394, error in=w398) -> (error out=w397:errorcluster)  [unwired: 1 in, 2 out]
      }
      frame "Add Package Extra Files" {
        # "Copy extra files"
        n231 = Current VI's Path() -> (path=w496:path)
        n232 = Strip Path(path=w496) -> (stripped path=w494:path)  [unwired: 1 out]
        n233 = property class="App"() -> ("App.Dir"=w488:path)  [unwired: 2 in, 2 out]
        n234 = Build Path(base path=w494, name or relative path="vipm-files") -> (appended path=w471:path)
        n235 = Unbundle By Name(w492) -> ("BuildPath"=w477:path)
        n236 = Build Path(base path=w488, name or relative path="LICENSE") -> (appended path=w486:path)
        n237 = Build Path(base path=w471, name or relative path="icon.bmp") -> (appended path=w491:path)
        n238 = Build Path(base path=w471, name or relative path="PreInstall.vi") -> (appended path=w475:path)
        n239 = Build Path(base path=w471, name or relative path="PostInstall.vi") -> (appended path=w469:path)
        n240 = Build Path(base path=w471, name or relative path="PreUninstall.vi") -> (appended path=w468:path)
        n241 = Build Path(base path=w471, name or relative path="PostUninstall.vi") -> (appended path=w467:path)
        n242 = Copy(8:w490, 9:TRUE ("overwrite (F)"), 10:w477, 11:w491) -> (0:w489:errorcluster)  [unwired: 1 in, 2 out]
        n243 = Copy(8:w489, 10:w477, 11:w486) -> (0:w481:errorcluster)  [unwired: 2 in, 2 out]
        n244 = Copy(8:w481, 9:TRUE ("overwrite (F)"), 10:w477, 11:w475) -> (0:w480:errorcluster)  [unwired: 1 in, 2 out]
        n245 = Copy(8:w480, 9:TRUE ("overwrite (F)"), 10:w477, 11:w469) -> (0:w479:errorcluster)  [unwired: 1 in, 2 out]
        n246 = Copy(8:w479, 9:TRUE ("overwrite (F)"), 10:w477, 11:w468) -> (0:w478:errorcluster)  [unwired: 1 in, 2 out]
        n247 = Copy(8:w478, 9:TRUE ("overwrite (F)"), 10:w477, 11:w467) -> (0:w470:errorcluster)  [unwired: 1 in, 2 out]
        n248 = Build Path(base path=w477, name or relative path="File Group 0") -> (appended path=w484:path)
        n249 = Create Folder(path (use dialog)=w484, error in=w470) -> (error out=w483:errorcluster)  [unwired: 1 in, 2 out]
      }
      frame "Copy Source To LabVIEW Versions" {
        # "Copy source files to all LV version selected"
        n250 = Unbundle By Name(w504) -> ("SourceFiles"=w499:path[], "LvVersion"=w502:path[])
        n251 = local read "LV_Versions"() -> (w503:cluster{"LvVersion":string, "Check":bool}[])
        n252 = property class="App"() -> ("App.Dir"=w498:path)  [unwired: 2 in, 2 out]
        n253 = for {
          tunnel: w503 -> [w515] mode=indexing
          tunnel: w502 -> [w507] mode=indexing
          shift-right: [w510] -> w500
          shift-left: w501 -> [w511]
          tunnel: w499 -> [w509]
          tunnel: w498 -> [w508]
          i -> [w513]
          n254 = Unbundle(w515) -> ("LvVersion"=w506:string, "Check"=w505:bool)
          n255 = Greater Than 0?(x=w513) -> (x > 0?=w512:bool)
          n256 = And(x=w505, y=w512) -> (x .and. y?=w514:bool)
          n257 = case shown="True" w514 {
            tunnel: w511 -> [w516 w526]
            tunnel: [w516 w525] -> w510
            tunnel: w509 -> [_ w529]
            tunnel: w508 -> [_ w528]
            tunnel: w507 -> [_ w527]
            tunnel: w506 -> [_ w519]
            frame False {
            }
            frame True {
              n258 = for {
                N -> [w537]
                tunnel: w529 -> [w550] mode=indexing
                tunnel: w528 -> [w551]
                tunnel: w527 -> [w549]
                shift-right: [w530] -> w525
                shift-left: w526 -> [w546]
                i -> [w538]
                stop <- w530 stop-if-true
                n259 = call <vilib>:"Compare Two Paths.vi"("Path 2"=w550, "Path 1"=w551) -> ("Relative Path from 1 to 2"=w548:path)  [unwired: 6 in, 3 out]
                n260 = Build Path(base path=w549, name or relative path=w548) -> (appended path=w544:path)
                n261 = Divide(x=w538, y=w537) -> (x/y=w536:dbl)
                n262 = Strip Path(path=w544) -> (stripped path=w547:path)  [unwired: 1 out]
                n263 = Multiply(x=w536, y=100.0) -> (x*y=→"Progress":dbl)
                n264 = call <vilib>:"Create Directory Recursive.vi"("error in (no error)"=w546, "directory"=w547) -> ("error out"=w545:errorcluster)  [unwired: 3 in, 2 out]
                n265 = call <vilib>:"Check if File or Folder Exists.vi"("error in (no error)"=w545, "path"=w544) -> ("error out"=w543:errorcluster, "file or folder exists?"=w540:bool, "dup path"=w542:path)  [unwired: 7 in]
                n266 = case shown="True" w540 {
                  tunnel: w543 -> [w552 w556]
                  tunnel: w542 -> [_ w555]
                  tunnel: [w552 w553] -> w541
                  frame False {
                  }
                  frame True {
                    n267 = Set Permissions(7:i16 511 ("permissions"), 8:w556, 11:w555) -> (0:w553:errorcluster)  [unwired: 2 in, 1 out]
                  }
                }
                n268 = Copy(8:w541, 9:TRUE ("overwrite (F)"), 10:w544, 11:w550) -> (0:w531:errorcluster, 3:w532:path)  [unwired: 1 in, 1 out]
                n269 = Set Permissions(7:i16 511 ("permissions"), 8:w531, 11:w532) -> (0:w530:errorcluster)  [unwired: 2 in, 1 out]
              }
              n270 = Format Date/Time String(time format string (%c)="%H:%M:%S") -> (date/time string=w517:string)  [unwired: 2 in]
              n271 = local read "Progress"() -> (w523:string)
              n272 = Format Into String(format string="Copy Files to: %s", initial string=w517, w519) -> (resulting string=w520:string)  [unwired: 1 in, 1 out]
              n273 = Concatenate Strings(w520, "\n" ("string"), w523) -> (w524:string)
              n274 = local write "Progress"(w524) -> ()
            }
          }
        }
      }
      frame "Copy Installer VI to Build Folder" {
        # "Copy and modify Installer VI"
        n275 = Current VI's Path() -> (path=w583:path)
        n276 = Strip Path(path=w583) -> (stripped path=w582:path)  [unwired: 1 out]
        n277 = local read "Output Folder"() -> (w557:path)
        n278 = Strip Path(path=w582) -> (stripped path=w581:path)  [unwired: 1 out]
        n279 = Build Path(base path=w581, name or relative path="Installer") -> (appended path=w579:path)
        n280 = Build Path(base path=w557, name or relative path="Installer.vi") -> (appended path=w558:path)
        n281 = Build Path(base path=w579, name or relative path="OpenGDS_Installer.vi") -> (appended path=w577:path)
        n282 = Open VI Reference(vi path=w577, error in (no error)=w560) -> (vi reference=w576:refnum<vi>, error out=w575:errorcluster)  [unwired: 4 in]
        n283 = invoke class="VI" method="Save.Instrument"(reference=w576, error in=w575, "Path to saved file"=w558) -> (reference out=w572:refnum<vi>, error out=w573:errorcluster)  [unwired: 3 in, 4 out]
        n284 = Bundle By Name(cluster=w584, "InstallerCopy"=w558) -> (w559:T1)
        n285 = call <vilib>:"Traverse for GObjects.vi"("Traverse Target"=TRef_TravTarget."BD", "error in (no error)"=w573, "Class Name"="EnumConstant", "VI Refnum"=w572) -> ("error out"=w568:errorcluster, "References"=w569:refnum<vi>[], "dup VI Refnum"=w564:refnum<vi>)  [unwired: 4 in, 1 out]
        n286 = for {
          tunnel: w569 -> [w595] mode=indexing
          shift-right: [w587] -> w567
          shift-left: w568 -> [w593]
          tunnel: [w586] -> w566 mode=indexing
          w594 = refnum<vi> refnum  # EnumConstant
          n287 = To More Specific Class(target class=w594, reference=w595, error in=w593) -> (specific class reference=w590:refnum<vi>, error out=w592:errorcluster)
          n288 = property class="EnmCnst"(reference=w590, error in=w592) -> (reference out=w589:refnum<vi>, error out=w591:errorcluster, "Typedef?"=w588:T6)
          n289 = case shown="\"typedef\", \"strict typedef\"" w588 {
            tunnel: w591 -> [w597 w601]
            tunnel: w589 -> [w596 w600]
            tunnel: [w597 w599] -> w587
            tunnel: [w596 w598] -> w586
            frame "not a typedef", Default {
            }
            frame "typedef", "strict typedef" {
              n290 = invoke class="EnmCnst" method="Discon Typedef"(reference=w600, error in=w601) -> (reference out=w598:refnum<vi>, error out=w599:errorcluster)  [unwired: 1 in, 1 out]
            }
          }
        }
        n291 = Close Reference(reference=w566, error in (no error)=w567) -> (error out=w565:errorcluster)
        n292 = invoke class="VI" method="Save.Instrument"(reference=w564, error in=w565) -> (reference out=w562:refnum<vi>, error out=w563:errorcluster)  [unwired: 4 in, 4 out]
        n293 = Close Reference(reference=w562, error in (no error)=w563) -> (error out=w561:errorcluster)
      }
      frame "Create Build Process" {
        # "Queue up the state machine"
        n294 = local read "LV_Versions"() -> (w610:cluster{"LvVersion":string, "Check":bool}[])
        n295 = Unbundle By Name(w609) -> ("LvVersion"=w608:path[])
        n296 = for {
          tunnel: w610 -> [w626] mode=indexing
          tunnel: w608 -> [_] mode=indexing
          tunnel: [w616] -> w607 mode=indexing if=w615
          tunnel: [w612] -> w602 mode=indexing
          i -> [w620]
          n297 = Unbundle By Name(w626) -> ("Check"=w621:bool, "LvVersion"=w624:string)
          n298 = Equal To 0?(x=w620) -> (x = 0?=w619:bool)
          n299 = Or(x=w619, y=w621) -> (x .or. y?=w615:bool)
          n300 = Search and Replace String(input string=w624, search string="LabVIEW ", replace string="LV" ("replace string (\"\")")) -> (result string=w612:string)  [unwired: 5 in, 3 out]
          n301 = case shown="False" w619 {
            tunnel: [w628 _] -> w618
            tunnel: w612 -> [w627 _]
            frame False {
              n302 = Format Into String(format string="Mass Compile>>%s\n", w627) -> (resulting string=w628:string)  [unwired: 2 in, 1 out]
            }
            frame True {
            }
          }
          n303 = Format Into String(format string="Copy Files to Package>>%s\nUpdate Spec File>>%s\nCreate Package File>>%s\nCreate ReadMe File>>%s\nZip Installation>>%s\n", w612, w612, w612, w612, w612) -> (resulting string=w617:string)  [unwired: 2 in, 1 out]
          n304 = Format Into String(format string="Update Installer>>%s\n", w612) -> (resulting string=w613:string)  [unwired: 2 in, 1 out]
          n305 = Concatenate Strings(w613, w618, w617) -> (w616:string)
        }
        n306 = Bundle By Name(cluster=w609, "LvVersion"=w602) -> (w603:T1)
        n307 = Build Array (concatenate)(w607, "CleanUpFolder\nDone") -> (w606:string[])
        n308 = Concatenate Strings(w606) -> (w604:string)
      }
      frame "------------------------------------" {
      }
      frame "Update Installer" {
        # "Update Installer"
        n309 = Unbundle By Name(w680) -> ("InstallerCopy"=w678:path, "VersionName"=w641:string)
        n310 = local read "Output Folder"() -> (w677:path)
        n311 = Format Into String(format string="Installer_OpenGDS_%s_%s.vi", w641, w633) -> (resulting string=w672:string)  [unwired: 2 in, 1 out]
        n312 = Build Path(base path=w677, name or relative path=w672) -> (appended path=w676:path)
        n313 = Format Into String(format string="OpenGDS_%s_%s.vip", w641, w633) -> (resulting string=w659:string)  [unwired: 2 in, 1 out]
        n314 = Format Into String(format string="ogds%s", w633) -> (resulting string=w639:string)  [unwired: 2 in, 1 out]
        n315 = Copy(8:w674, 9:TRUE ("overwrite (F)"), 10:w676, 11:w678) -> (0:w671:errorcluster, 3:w656:path)  [unwired: 1 in, 1 out]
        n316 = property class="App"() -> ("App.Dir"=w652:path)  [unwired: 2 in, 2 out]
        n317 = Open VI Reference(vi path=w656, error in (no error)=w671) -> (vi reference=w662:refnum<vi>, error out=w663:errorcluster)  [unwired: 4 in]
        n318 = call <vilib>:"Traverse for GObjects.vi"("Traverse Target"=TRef_TravTarget."BD", "error in (no error)"=w663, "Class Name"="StringConstant", "VI Refnum"=w662) -> ("error out"=w668:errorcluster, "References"=w669:refnum<vi>[], "dup VI Refnum"=w637:refnum<vi>)  [unwired: 4 in, 1 out]
        n319 = Build Path(base path=w652, name or relative path="LICENSE") -> (appended path=w650:path)
        n320 = Format Into String(format string="OpenGDS %s", w641) -> (resulting string=w642:string)  [unwired: 2 in, 1 out]
        n321 = for {
          tunnel: w669 -> [w711] mode=indexing
          shift-right: [w703] -> w667
          shift-left: w668 -> [w709]
          tunnel: [w702] -> w666 mode=indexing
          tunnel: w659 -> [w701]
          tunnel: w642 -> [w700]
          tunnel: w639 -> [w699]
          w710 = refnum<vi> refnum  # StringConstant
          n322 = To More Specific Class(target class=w710, reference=w711, error in=w709) -> (specific class reference=w706:refnum<vi>, error out=w708:errorcluster)
          n323 = property class="StrCnst"(reference=w706, error in=w708) -> (reference out=w705:refnum<vi>, error out=w707:errorcluster, "Label.Text"=w704:string)
          n324 = case shown="\"TempFolderName\"" w704 {
            tunnel: w707 -> [w713 w718 w723 w728]
            tunnel: w705 -> [w712 w717 w722 w727]
            tunnel: [w713 w716 w721 w726] -> w703
            tunnel: [w712 w715 w720 w725] -> w702
            tunnel: w701 -> [_ w714 _ _]
            tunnel: w700 -> [_ _ _ w724]
            tunnel: w699 -> [_ _ w719 _]
            frame Default {
            }
            frame "VIP-File" {
              n325 = property class="StrCnst"(reference=w717, error in=w718, "Value"=w714) -> (reference out=w715:refnum<vi>, error out=w716:errorcluster)
            }
            frame "TempFolderName" {
              n326 = property class="StrCnst"(reference=w722, error in=w723, "Value"=w719) -> (reference out=w720:refnum<vi>, error out=w721:errorcluster)
            }
            frame "Version" {
              n327 = property class="StrCnst"(reference=w727, error in=w728, "Value"=w724) -> (reference out=w725:refnum<vi>, error out=w726:errorcluster)
            }
          }
        }
        n328 = Read from Text File(file (use dialog)=w650) -> (text=w649:string)  [unwired: 3 in, 3 out]
        n329 = Bundle By Name(cluster=w680, "InstallerFile"=w656) -> (w657:T1)
        n330 = Close Reference(reference=w666, error in (no error)=w667) -> (error out=w654:errorcluster)
        n331 = call <vilib>:"Traverse for GObjects.vi"("Traverse Target"=TRef_TravTarget."FP", "error in (no error)"=w654, "Class Name"="String", "VI Refnum"=w637) -> ("error out"=w644:errorcluster, "References"=w645:refnum<vi>[])  [unwired: 4 in, 2 out]
        n332 = for {
          tunnel: w645 -> [w691] mode=indexing
          shift-right: [w683] -> w648
          shift-left: w644 -> [w689]
          tunnel: [w682] -> w647 mode=indexing
          tunnel: w649 -> [w681]
          w690 = refnum<vi> refnum  # String
          n333 = To More Specific Class(target class=w690, reference=w691, error in=w689) -> (specific class reference=w686:refnum<vi>, error out=w688:errorcluster)
          n334 = property class="Str"(reference=w686, error in=w688) -> (reference out=w685:refnum<vi>, error out=w687:errorcluster, "Label.Text"=w684:string)
          n335 = case shown="\"Lic\"" w684 {
            tunnel: w687 -> [w693 w698]
            tunnel: w685 -> [w692 w697]
            tunnel: [w693 w696] -> w683
            tunnel: [w692 w694] -> w682
            tunnel: w681 -> [_ w695]
            frame Default {
            }
            frame "Lic" {
              n336 = property class="Str"(reference=w697, error in=w698, "Value"=w695) -> (reference out=w694:refnum<vi>, error out=w696:errorcluster)
            }
          }
        }
        n337 = Close Reference(reference=w647, error in (no error)=w648) -> (error out=w646:errorcluster)
        n338 = invoke class="VI" method="Default Vals.Make Curr Default"(reference=w637, error in=w646) -> (error out=w635:errorcluster)  [unwired: 1 in, 2 out]
        n339 = property class="VI"(reference=w637, error in=w635, "Exec.RunOnOpen"=TRUE ("Execution:Run When Opened")) -> (reference out=w636:refnum<vi>, error out=w638:errorcluster)
        n340 = invoke class="VI" method="Save.Instrument"(reference=w636, error in=w638) -> (reference out=w664:refnum<vi>, error out=w665:errorcluster)  [unwired: 4 in, 4 out]
        n341 = Close Reference(reference=w664, error in (no error)=w665) -> (error out=w658:errorcluster)
      }
      frame "Mass Compile" {
        # "\"C:\\Program Files\\National Instruments\\LabVIEW 2013\\LabVIEW.exe\" \"C:\\Program Files (x86)\\National Instruments\\LabVIEW 2012\\Open_GDS_Tools\\Build_Release\\BuildRelease_SubVIs\\BuildRelease_RecompileOpenGDS.vi\" -- \"2120\" \"C:\\...\\spec\""
        # "Mass Compile"
        n342 = Unbundle By Name(w764) -> ("SourceFiles"=w754:path[], "LvVersion"=w773:path[], "LvVersion"=w775:string[])
        n343 = Unbundle By Name(w764) -> ("BuildPath"=w742:path, "SpecFile"=w763:path, "InstallerFile"=w741:path, "LogFolder"=w740:path, "IniFiles"=w758:path[])
        n344 = vi-ref "BuildRelease_RecompileOpenGDS_RemoveDebugFlag.vi"() -> (w733:refnum<vi>)
        n345 = vi-ref "BuildRelease_RecompileOpenGDS.vi"() -> (w769:refnum<vi>)
        n346 = property class="VI"(reference=w769, error in=w729) -> (error out=w766:errorcluster, "Path"=w767:path)  [unwired: 1 out]
        n347 = property class="VI"(reference=w733, error in=w729) -> (error out=w736:errorcluster, "Path"=w735:path)  [unwired: 1 out]
        n348 = Search 1D Array(1D array=w775, element=w774) -> (index of element=w772:i32)  [unwired: 1 in]
        n349 = local read "Output Folder"() -> (w762:path)
        n350 = Set Permissions(7:i16 365 ("permissions"), 8:w766, 11:w767) -> (0:w731:errorcluster, 3:w765:path)  [unwired: 2 in]
        n351 = Set Permissions(7:i16 365 ("permissions"), 8:w736, 11:w735) -> (0:w732:errorcluster)  [unwired: 2 in, 1 out]
        n352 = Index Array(array=w773, index=w772) -> (element=w738:path)
        n353 = Merge Errors(w731, w732) -> (w730:errorcluster)
        n354 = Build Path(base path=w762, name or relative path="TempFolder") -> (appended path=w760:path)
        n355 = for {
          shift-right: [w801] -> w744
          shift-left: w730 -> [w802]
          tunnel: w758 -> [w797] mode=indexing
          tunnel: w760 -> [w800]
          tunnel: [w798] -> w759 mode=indexing
          tunnel: w738 -> [w796]
          tunnel: [w795] -> w737 mode=indexing
          # "Remove ini files\nbefore starting LV"
          n356 = Build Path(base path=w796, name or relative path=w797) -> (appended path=w795:path)
          n357 = Move(source path=w795, error in=w802, 9:TRUE ("overwrite (F)"), 10:w800) -> (error out=w801:errorcluster, 3:w798:path)  [unwired: 1 in, 1 out]
        }
        n358 = Current VI's Path() -> (path=w746:path)
        n359 = Strip Path(path=w746) -> (stripped path=w739:path)  [unwired: 1 out]
        n360 = Format Into String(format string="\"%s\\\\LabVIEW.exe\" \"%s\" -- \"%s\" \"%s\" \"%s\" \"%s\"", w738, w765, w742, w763, w741, w740) -> (resulting string=w770:string)  [unwired: 2 in, 1 out]
        n361 = Build Path(base path=w739, name or relative path="vipm-files") -> (appended path=w751:path)
        n362 = for {
          tunnel: w754 -> [w787] mode=indexing
          tunnel: w738 -> [w789]
          tunnel: [w788] -> w753 mode=indexing
          n363 = Path To String(path=w787) -> (string=w786:string)
          n364 = Match Pattern(string=w786, regular expression="LabVIEW [0-9]+\\\\") -> (after substring=w784:string)  [unwired: 1 in, 3 out]
          n365 = Build Path(base path=w789, name or relative path=w784) -> (appended path=w788:path)
        }
        n366 = Build Array("PreInstall.vi" ("name or relative path"), "PostInstall.vi" ("name or relative path"), "PreUninstall.vi" ("name or relative path"), "PostUninstall.vi" ("name or relative path")) -> (w752:string[])
        n367 = for {
          tunnel: w751 -> [w783]
          tunnel: w752 -> [w782] mode=indexing
          shift-right: [w779] -> w743
          shift-left: w744 -> [w780]
          tunnel: w742 -> [w777]
          n368 = Build Path(base path=w783, name or relative path=w782) -> (appended path=w781:path)
          n369 = Copy(8:w780, 9:TRUE ("overwrite (F)"), 10:w777, 11:w781) -> (0:w779:errorcluster)  [unwired: 1 in, 2 out]
        }
        n370 = call <vilib>:"System Exec.vi"("error in (no error)"=w743, "command line"=w770) -> ("error out"=w757:errorcluster)  [unwired: 6 in, 3 out]
        n371 = Bundle By Name(cluster=w764, "SourceFiles"=w753) -> (w755:T1)
        n372 = for {
          shift-right: [w793] -> w756
          shift-left: w757 -> [w794]
          tunnel: w759 -> [w792] mode=indexing
          tunnel: w737 -> [w791] mode=indexing
          # "Restore ini files"
          n373 = Move(source path=w792, error in=w794, 9:TRUE ("overwrite (F)"), 10:w791) -> (error out=w793:errorcluster)  [unwired: 1 in, 2 out]
        }
      }
      frame "Update Spec File" {
        (unwired) "%sExclusive_LabVIEW_Version=\">=%s.0\"%s" ("format string")
        # "\"C:\\Program Files\\National Instruments\\LabVIEW 2013\\LabVIEW.exe\" \"C:\\Program Files (x86)\\National Instruments\\LabVIEW 2012\\Open_GDS_Tools\\Build_Release\\BuildRelease_SubVIs\\BuildRelease_RecompileOpenGDS.vi\" -- \"2120\" \"C:\\...\\spec\""
        # "Mass Compile"
        n374 = Unbundle By Name(w819) -> ("LvVersion"=w821:path[], "LvVersion"=w823:string[])  [unwired: 1 out]
        n375 = Unbundle By Name(w819) -> ("BuildPath"=w817:path)
        n376 = Search 1D Array(1D array=w823, element=w822) -> (index of element=w820:i32)  [unwired: 1 in]
        n377 = Build Path(base path=w817, name or relative path="spec") -> (appended path=w804:path)
        n378 = Index Array(array=w821, index=w820) -> (element=w808:path)
        n379 = Path To String(path=w808) -> (string=w807:string)
        n380 = Read from Text File(file (use dialog)=w804, error in=w818) -> (text=w814:string, error out=w815:errorcluster)  [unwired: 2 in, 2 out]
        n381 = Match Pattern(string=w807, regular expression="[0-9][0-9]$") -> (match substring=w805:string)  [unwired: 1 in, 3 out]
        n382 = Match Pattern(string=w814, regular expression="Exclusive_LabVIEW_Version=\"[~\"]+\"") -> (before substring=w812:string, after substring=w811:string)  [unwired: 1 in, 2 out]
        n383 = Format Into String(format string="%sExclusive_LabVIEW_Version=\"=%s.0\"%s", w812, w805, w811) -> (resulting string=w810:string)  [unwired: 2 in, 1 out]
        n384 = Write to Text File(file (use dialog)=w804, text=w810, error in=w815) -> (error out=w803:errorcluster)  [unwired: 1 in, 2 out]
      }
      frame "Copy Files to Package" {
        # "Copy Source files"
        n385 = Unbundle By Name(w826) -> ("BuildPath"=w839:path, "SourceFiles"=w837:path[])
        n386 = Unbundle By Name(w826) -> ("LvVersion"=w831:path[], "LvVersion"=w833:string[])
        n387 = Search 1D Array(1D array=w833, element=w830) -> (index of element=w832:i32)  [unwired: 1 in]
        n388 = Index Array(array=w831, index=w832) -> (element=w829:path)
        n389 = Build Path(base path=w839, name or relative path="File Group 0") -> (appended path=w828:path)
        n390 = call <vilib>:"Create Directory Recursive.vi"("directory"=w828) -> ("directory copy"=w827:path)  [unwired: 4 in, 2 out]
        n391 = for {
          N -> [w857]
          tunnel: w837 -> [w848] mode=indexing
          tunnel: w829 -> [w862]
          shift-right: [w850] -> w835
          shift-left: w836 -> [w861]
          tunnel: w827 -> [w859]
          tunnel: [w849] -> w825 mode=indexing if=w851
          i -> [w858]
          stop <- w850 stop-if-true
          n392 = Increment(x=w858) -> (x+1=w840:i32)
          n393 = call <vilib>:"Compare Two Paths.vi"("error in (no error)"=w861, "Path 2"=w848, "Path 1"=w862) -> ("error out"=w844:errorcluster, "Relative Path from 1 to 2"=w860:path)  [unwired: 5 in, 2 out]
          n394 = Divide(x=w840, y=w857) -> (x/y=w841:dbl)
          n395 = Build Path(base path=w859, name or relative path=w860) -> (appended path=w845:path)
          n396 = Multiply(x=w841, y=100) -> (x*y=w855:dbl)
          n397 = Strip Path(path=w845) -> (stripped path=w842:path)  [unwired: 1 out]
          n398 = local write "Progress"(w855) -> ()
          n399 = call <vilib>:"Create Directory Recursive.vi"("error in (no error)"=w844, "directory"=w842) -> ("error out"=w843:errorcluster)  [unwired: 3 in, 2 out]
          n400 = File/Directory Info(path=w848, error in=w843) -> (directory=w846:bool, error out=w847:errorcluster)  [unwired: 5 out]
          n401 = case shown="False" w846 {
            tunnel: [w869 w870] -> w850
            tunnel: w845 -> [w866 _]
            tunnel: [w865 _] -> w849
            tunnel: w848 -> [w864 _]
            tunnel: w847 -> [w863 w870]
            frame False {
              n402 = Set Permissions(7:i16 511 ("permissions"), 11:w866) -> (3:w865:path)  [unwired: 3 in, 1 out]
              n403 = Copy(8:w863, 9:TRUE ("overwrite (F)"), 10:w865, 11:w864) -> (0:w869:errorcluster)  [unwired: 1 in, 2 out]
            }
            frame True {
            }
          }
          n404 = Strip Path(path=w849) -> (name=w854:string)  [unwired: 1 out]
          n405 = Match Pattern(string=w854, regular expression="^GOOP_[A-Za-z]+.ini$") -> (offset past match=w852:i32)  [unwired: 1 in, 3 out]
          n406 = Greater Or Equal To 0?(x=w852) -> (x >= 0?=w851:bool)
        }
      }
      frame "Create Package File" {
        # "Copy extra files"
        n407 = Unbundle By Name(w890) -> ("BuildPath"=w874:path, "VersionName"=w873:string)
        n408 = local read "Output Folder"() -> (w881:path)
        n409 = call <vilib>:"Recursive File List.vi"("error in (no error)"=w889, "Folder Path"=w874) -> ("error out"=w882:errorcluster, "All Files in Dir"=w883:path[])  [unwired: 5 in, 3 out]
        n410 = Format Into String(format string="OpenGDS_%s_%s.vip", w873, w879) -> (resulting string=w878:string)  [unwired: 2 in, 1 out]
        n411 = Build Path(base path=w881, name or relative path=w878) -> (appended path=w871:path)
        n412 = Bundle By Name(cluster=w890, "VIP-File"=w871) -> (w872:T1)
        n413 = Delete(path (use dialog)=w871) -> (deleted path=w876:path)  [unwired: 4 in, 2 out]
        n414 = call <vilib>:"New Zip File.vi"("error in (no error)"=w882, "confirm overwrite? (F)"=TRUE, "target"=w876) -> ("error out"=w886:errorcluster, "zip file out"=w887:i64)  [unwired: 2 in, 1 out]
        n415 = for {
          N -> [w894]
          tunnel: w883 -> [w899] mode=indexing
          shift-right: [w901] -> w884
          shift-left: w887 -> [w903]
          shift-right: [w893] -> w885
          shift-left: w886 -> [w902]
          tunnel: w874 -> [w900]
          i -> [w895]
          stop <- w893 stop-if-true
          n416 = Increment(x=w895) -> (x+1=w891:i32)
          n417 = Divide(x=w891, y=w894) -> (x/y=w892:dbl)
          n418 = call <vilib>:"Compare Two Paths.vi"("Path 2"=w899, "Path 1"=w900) -> ("Relative Path from 1 to 2"=w898:path)  [unwired: 6 in, 3 out]
          n419 = Multiply(x=w892, y=100) -> (x*y=w896:dbl)
          n420 = call <vilib>:"Add File to Zip.vi"("error in (no error)"=w902, "destination path in zip"=w898, "source file path"=w899, "zip file in"=w903) -> ("error out"=w893:errorcluster, "zip file out"=w901:i64)  [unwired: 6 in]
          n421 = local write "Progress"(w896) -> ()
        }
        n422 = call <vilib>:"Close Zip File.vi"("error in (no error)"=w885, "zip file in"=w884) -> ("error out"=w877:errorcluster)  [unwired: 5 in]
      }
      frame "Create ReadMe File" {
        # "Update Installer"
        n423 = Unbundle By Name(w918) -> ("InstallerFile"=w905:path, "VersionName"=w907:string)
        n424 = local read "Output Folder"() -> (w916:path)
        n425 = Strip Path(path=w905) -> (name=w904:string)  [unwired: 1 out]
        n426 = Format Into String(format string="ReadMe_OpenGDS_%s_%s.txt", w907, w906) -> (resulting string=w914:string)  [unwired: 2 in, 1 out]
        n427 = Build Path(base path=w916, name or relative path=w914) -> (appended path=w912:path)
        n428 = Format Into String(format string="Welcome to OpenGDS\nThis is the release: %s, build for: %s\nTo install this version use either, VIPM or the installer VI (%s)." ("text"), w907, w906, w904) -> (resulting string=w908:string)  [unwired: 2 in, 1 out]
        n429 = Bundle By Name(cluster=w918, "ReadMeFile"=w912) -> (w913:T1)
        n430 = Write to Text File(file (use dialog)=w912, text=w908, error in=w911) -> (error out=w910:errorcluster)  [unwired: 1 in, 2 out]
      }
      frame "Zip Installation" {
        # "Zip Installtion"
        n431 = Unbundle By Name(w920) -> ("VIP-File"=w926:path, "ReadMeFile"=w925:path, "InstallerFile"=w924:path)
        n432 = Unbundle By Name(w920) -> ("VersionName"=w919:string)
        n433 = local read "Output Folder"() -> (w921:path)
        n434 = Format Into String(format string="OpenGDS_%s_%s.zip", w919, w932) -> (resulting string=w931:string)  [unwired: 2 in, 1 out]
        n435 = Build Array(w926, w925, w924) -> (w922:path[])
        n436 = Build Path(base path=w921, name or relative path=w931) -> (appended path=w929:path)
        n437 = Delete(path (use dialog)=w929) -> (deleted path=w928:path)  [unwired: 4 in, 2 out]
        n438 = call <vilib>:"New Zip File.vi"("error in (no error)"=w923, "confirm overwrite? (F)"=TRUE, "target"=w928) -> ("error out"=w936:errorcluster, "zip file out"=w937:i64)  [unwired: 2 in, 1 out]
        n439 = for {
          N -> [w942]
          tunnel: w922 -> [w947] mode=indexing
          shift-right: [w949] -> w934
          shift-left: w937 -> [w951]
          shift-right: [w941] -> w935
          shift-left: w936 -> [w950]
          tunnel: w921 -> [w948]
          i -> [w943]
          stop <- w941 stop-if-true
          n440 = Increment(x=w943) -> (x+1=w939:i32)
          n441 = Divide(x=w939, y=w942) -> (x/y=w940:dbl)
          n442 = call <vilib>:"Compare Two Paths.vi"("Path 2"=w947, "Path 1"=w948) -> ("Relative Path from 1 to 2"=w946:path)  [unwired: 6 in, 3 out]
          n443 = Multiply(x=w940, y=100) -> (x*y=w944:dbl)
          n444 = call <vilib>:"Add File to Zip.vi"("error in (no error)"=w950, "destination path in zip"=w946, "source file path"=w947, "zip file in"=w951) -> ("error out"=w941:errorcluster, "zip file out"=w949:i64)  [unwired: 6 in]
          n445 = local write "Progress"(w944) -> ()
        }
        n446 = call <vilib>:"Close Zip File.vi"("error in (no error)"=w935, "zip file in"=w934) -> ("error out"=w930:errorcluster)  [unwired: 5 in]
      }
      frame "CleanUpFolder" {
        n447 = local read "Output Folder"() -> (w956:path)
        n448 = Build Path(base path=w956, name or relative path="TempFolder") -> (appended path=w960:path)
        n449 = List Folder(path=w956, pattern="*.txt" ("name or relative path")) -> (path out=w954:path, filenames=w955:string[])  [unwired: 2 in, 2 out]
        n450 = List Folder(path=w956, pattern="*.vi" ("name or relative path")) -> (path out=w953:path, filenames=w952:string[])  [unwired: 2 in, 2 out]
        n451 = for {
          tunnel: w955 -> [w970] mode=indexing
          tunnel: w954 -> [w969]
          n452 = Build Path(base path=w969, name or relative path=w970) -> (appended path=w968:path)
          n453 = Delete(path (use dialog)=w968) -> ()  [unwired: 4 in, 3 out]
        }
        n454 = for {
          tunnel: w952 -> [w967] mode=indexing
          tunnel: w953 -> [w966]
          n455 = Build Path(base path=w966, name or relative path=w967) -> (appended path=w965:path)
          n456 = Delete(path (use dialog)=w965) -> ()  [unwired: 4 in, 3 out]
        }
        n457 = Delete(path (use dialog)=w960, entire hierarchy (F)=TRUE) -> ()  [unwired: 3 in, 3 out]
      }
    }
    n458 = local write "Progress"(w14) -> ()
  }
